vi "RT Driver VI.vi"(7 "Operation":T1, 11 "Device Reference in":T2 format="%.0x") -> (0 "Error Code":i32)   [LabVIEW 2017, in "DSF Engine.lvlib"]
uses:
  DSF Engine.lvlib
  <vilib>/NI Veristand/Custom Device API/Custom Device Item Ref.ctl
  <vilib>/NI Veristand/Custom Device API/Hardware Interface Driver VI Operation.ctl
  VeriStand DSF/VeriStand DSF.lvclass
  DSF Core.lvlibp/Classes/Framework/Framework Options.ctl
  DSF Core.lvlibp/Typedefs/DSF FIFO Options.ctl
  DSF Core.lvlibp/Classes/Thread/DSF Thread Options.ctl
  DSF Core.lvlibp/Typedefs/DSF Plugin Options.ctl
  DSF Core.lvlibp/Typedefs/DSF Performance Options.ctl
  <vilib>/NI Veristand/Custom Device API/Global Data Refs.vi
  DSF Core.lvlibp/Classes/Framework/Increment Framework Cycle.vi
  DSF Core.lvlibp/Classes/Framework/Start of Cycle.vi
  DSF Core.lvlibp/Classes/Framework/Active Plugins.vi
  DSF Core.lvlibp/Classes/Framework/Receive.vi
  <vilib>/NI Veristand/Custom Device API/Custom Device API.lvlib
  DSF Core.lvlibp/Classes/Framework/Framework.lvclass
  DSF Core.lvlibp
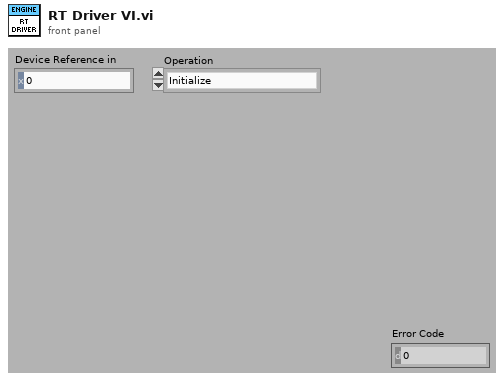
[diagram p1: front panel]
types:
  T1 = typedef "Custom Device API.lvlib/Hardware Interface Driver VI Operation.ctl" = enum16{"Initialize", "Start", "Read Data from HW", "Write Data to HW", "Close"}
  T2 = typedef "Custom Device API.lvlib/Custom Device Item Ref.ctl" = u64
  T3 = typedef "DSF Core.lvlibp/DSF Engine Framework Configuration.ctl" = cluster{"components directory":path, "Plugins":T4[]}
  T4 = typedef "DSF Core.lvlibp/DSF Engine Plugin Configuration.ctl" = cluster{"name":string, "components":string[], "cycle timing":T5, "threads":T6[], "Transfer Groups":T8[], "settings":T7}
  T5 = typedef "DSF Core.lvlibp/DSF Timing Info.ctl" = cluster{"priority":u64, "decimation":u64, "offset":u64}
  T6 = typedef "DSF Core.lvlibp/DSF Engine Plugin Thread Configuration.ctl" = cluster{"buffer converter settings":T7, "transceiver settings":T7, "processor":i32, "priority offset":i16}
  T7 = typedef "DSF Core.lvlibp/DSF Settings Info.ctl" = cluster{"key":string, "value":string}[]
  T8 = typedef "DSF Core.lvlibp/DSF Engine Transfer Group Configuration.ctl" = cluster{"name":string, "direction":T9, "cycle timing":T5, "thread index":i32, "settings":T7, "Transfers":T10[], "timeout behavior":T14}
  T9 = typedef "DSF Core.lvlibp/DSF Direction.ctl" = enum8{"Tx", "Rx"}
  T10 = typedef "DSF Core.lvlibp/DSF Engine Transfer Configuration.ctl" = cluster{"name":string, "byte order":T11, "settings":T7, "channels":T12[]}
  T11 = typedef "DSF Core.lvlibp/DSF Byte Order.ctl" = enum8{"big-endian", "little-endian"}
  T12 = typedef "DSF Core.lvlibp/DSF Engine Channel Configuration.ctl" = cluster{"string offset":u64, "string data type":T13, "engine data type":T13, "name":string, "settings":T7}
  T13 = typedef "DSF Core.lvlibp/DSF Data Type.ctl" = enum8{"Bool", "SGL", "DBL", "I8", "I16", "I32", "I64", "U8", "U16", "U32", "U64"}
  T14 = typedef "DSF Core.lvlibp/DSF Timeout Behavior.ctl" = enum8{"Increment Late Count", "Throw Error"}
  T15 = typedef "DSF Core.lvlibp/Framework.lvclass/Framework Options.ctl" = cluster{"FIFO Options":T16, "Thread Options":T17, "Plugin Options":T18, "Performance Options":T19}
  T16 = typedef "DSF Core.lvlibp/DSF FIFO Options.ctl" = cluster{"Infinite Timeouts":bool}
  T17 = typedef "DSF Core.lvlibp/DSF Thread Options.ctl" = cluster{"Show FP On Call":bool, "Close FP After Call":bool, "Allow Debugging":bool, "Show Menu Bar":bool, "Reposition Windows":bool}
  T18 = typedef "DSF Core.lvlibp/DSF Plugin Options.ctl" = cluster{"Default Components":bool}
  T19 = typedef "DSF Core.lvlibp/DSF Performance Options.ctl" = cluster{"Measure Period":bool, "Measure Rx/Tx Duration":bool}
  T20 = typedef "Custom Device API.lvlib/Data Table Ref.ctl" = cluster{"Ptr.Beg":u64, "Ptr.End":u64}
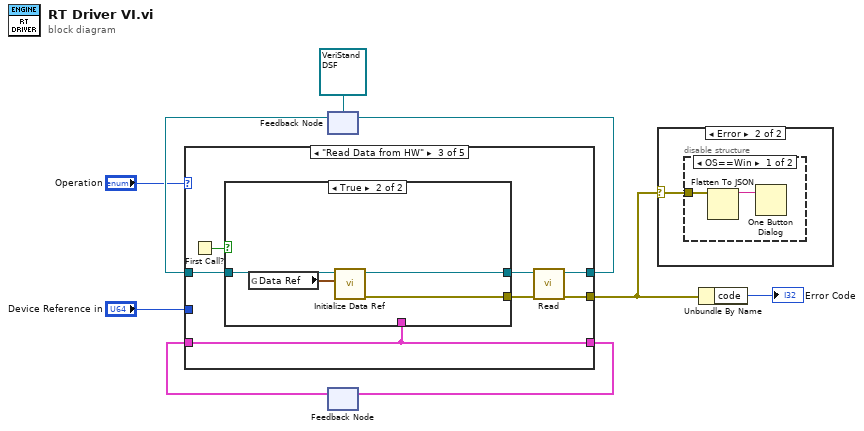
[diagram p0: block diagram]
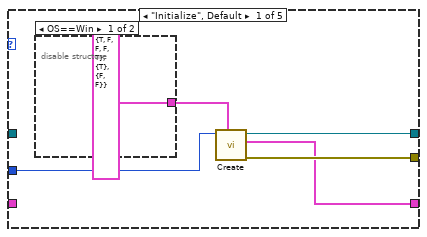
[diagram p4: hidden frame]
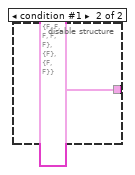
[diagram p5: hidden frame]
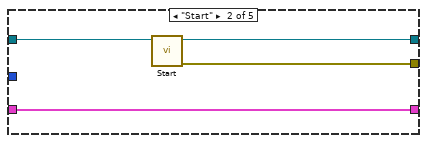
[diagram p6: hidden frame]
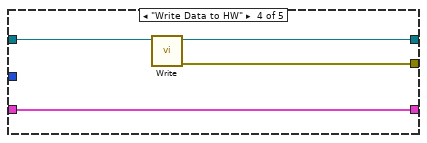
[diagram p8: hidden frame]
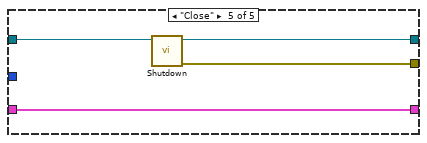
[diagram p9: hidden frame]
diagram:
  n1 = feedback #1(refnum<class "VeriStand DSF.lvclass"> refnum ("Data Sharing Framework Engine.lvlib:VeriStand Data Sharing Framework.lvclass")) -> (w9:refnum<class "VeriStand DSF.lvclass">)
  n2 = feedback #2() -> (w2:T3)  [unwired: 1 in]
  n3 = case shown="\"Read Data from HW\"" "Operation" {
    tunnel: [w11 w19 w25 w35 w38] -> w7
    tunnel: w9 -> [_ w20 w26 w36 w40]
    tunnel: "Device Reference in" -> [w13 _ _ _ _]
    tunnel: [w14 w18 w22 w34 w39] -> w3
    tunnel: [w10 w17 w21 w33 w37] -> w1
    tunnel: w2 -> [_ w17 w21 w33 w37]
    frame "Initialize", Default {
      n4 = disable-structure shown="OS==Win" {
        disable-tunnel: [T15 {"FIFO Options"={"Infinite Timeouts"=TRUE}, "Thread Options"={"Show FP On Call"=TRUE, "Close FP After Call"=FALSE, "Allow Debugging"=FALSE, "Show Menu Bar"=FALSE, "Reposition Windows"=TRUE}, "Plugin Options"={"Default Components"=TRUE}, "Performance Options"={"Measure Period"=FALSE, "Measure Rx/Tx Duration"=FALSE}} ("options") T15 {"FIFO Options"={"Infinite Timeouts"=FALSE}, "Thread Options"={"Show FP On Call"=FALSE, "Close FP After Call"=FALSE, "Allow Debugging"=FALSE, "Show Menu Bar"=FALSE, "Reposition Windows"=FALSE}, "Plugin Options"={"Default Components"=FALSE}, "Performance Options"={"Measure Period"=FALSE, "Measure Rx/Tx Duration"=FALSE}} ("options")] -> w12
        frame condition #0 (active) {
        }
        frame condition #1 {
        }
      }
      n5 = call "Create.vi"("options"=w12, "Device Item Ref"=w13) -> ("error out"=w14:errorcluster, "framework configuration"=w10:T3, "VeriStand Framework"=w11:refnum<class "VeriStand DSF.lvclass">)  [unwired: 7 in]
    }
    frame "Start" {
      n6 = call-dynamic "Start.vi"("VeriStand Data Sharing Framework in"=w20) -> ("error out"=w18:errorcluster, "VeriStand Data Sharing Framework out"=w19:refnum<class "VeriStand DSF.lvclass">)  [unwired: 9 in]
    }
    frame "Read Data from HW" {
      n7 = First Call?() -> (First Call?: T/F=w27:bool)
      n8 = case shown="True" w27 {
        tunnel: w26 -> [w28 w32]
        tunnel: [w28 w29] -> w24
        tunnel: [_ w30] -> w23
        tunnel: w21 -> [_ _]
        frame False {
        }
        frame True {
          n9 = global read "Global Data Refs.vi" "Data Ref"() -> (w31:T20)
          n10 = call "Initialize Data Ref.vi"("Data Ref"=w31, "VeriStand Data Sharing Framework in"=w32) -> ("error out"=w30:errorcluster, "VeriStand Data Sharing Framework out"=w29:refnum<class "VeriStand DSF.lvclass">)  [unwired: 8 in]
        }
      }
      n11 = call "Read.vi"("error in (no error)"=w23, "VeriStand DSF in"=w24) -> ("error out"=w22:errorcluster, "VeriStand DSF out"=w25:refnum<class "VeriStand DSF.lvclass">)  [unwired: 8 in]
    }
    frame "Write Data to HW" {
      n12 = call "Write.vi"("VeriStand Data Sharing Framework in"=w36) -> ("error out"=w34:errorcluster, "VeriStand Data Sharing Framework out"=w35:refnum<class "VeriStand DSF.lvclass">)  [unwired: 9 in]
    }
    frame "Close" {
      n13 = call-dynamic "Shutdown.vi"("VeriStand Data Sharing Framework in"=w40) -> ("error out"=w39:errorcluster, "VeriStand Data Sharing Framework out"=w38:refnum<class "VeriStand DSF.lvclass">)  [unwired: 9 in]
    }
  }
  n14 = feedback-in #1(w7) -> ()
  n15 = feedback-in #2(w1) -> ()
  n16 = case shown="Error" w3 {
    selector: w3 -> [_ w41]
    frame No Error {
    }
    frame Error {
      n17 = disable-structure shown="OS==Win" {
        disable-tunnel: w41 -> [w43 _]
        frame condition #0 (active) {
          n18 = Flatten To JSON(anything=w43) -> (JSON string=w42:string)  [unwired: 2 in, 1 out]
          n19 = One Button Dialog(message=w42) -> ()  [unwired: 1 in, 1 out]
        }
        frame condition #1 {
        }
      }
    }
  }
  n20 = Unbundle By Name(w3) -> ("code"=→"Error Code":i32)
